vi "Process.vi"(8 "error in":errorcluster, 11 "GUI":refnum<class "GUI.lvclass">) -> (0 "error out":errorcluster, 3 "GUI out":refnum<class "GUI.lvclass">)   [LabVIEW 2022 SP3, in "GUI.lvclass"]
doc: "---------------------------------------------------------------\nJKI State Machine Objects™\nhttp://jki.net/state-machine-objects/\nCopyright (C) 2005-2015, JKI <info@jki.net>\nALL RIGHTS RESERVEDJKI State Machine Objects (SMO) 1.0.0.5\nJKI - JKI\nCopyright (c) 2016, JKI"
uses:
  GUI.lvclass
  <vilib>/JKI/JKI SMO/SMO/SMO.lvclass
  <vilib>/JKI/JKI SMO/SMO/Typedefs/Parent Call--Enum.ctl
  Typedefs/Value.ctl
  <vilib>/JKI/JKI SMO/SMO.UI/SMO.UI.lvclass
  DB2/DB2.lvclass
  Analyzer/Analyzer.lvclass
  Home/Home.lvclass
  C:/Program Files (x86)/National Instruments/LabVIEW 2022/vi.lib/JKI/JKI SMO/SMO.UI/SMO.UI.lvclass
  C:/Program Files (x86)/National Instruments/LabVIEW 2022/vi.lib/JKI/JKI SMO/SMO/SMO.lvclass
  C:/Users/uib01493/Documents/CIS_580_Data_Analytics_in_SW_Eng/002_Source_Code/002_GUI/002_SRC/GUI/GUI.lvclass
panel:
  in  "Menu Btns":T1(radio) caption="Radio Btns"
  out "Status":string
  # "Software Requirements Tracing Tool (development)"
  # "For instructions on how to use the JKI State Machine Objects, examples and video tutorials, visit:\nhttp://jki.net/state-machine-objects/\n\nJKI State Machine Objects™\nhttp://jki.net/state-machine-objects/\nCopyright (C) 2005-2015, JKI <info@jki.net>\nALL RIGHTS RESERVED"
types:
  T1 = enum32{"Home", "Analyzer", "Button 3", "Settings"}
  T2 = typedef "SMO.lvclass/Parent Call--Enum.ctl" = enum16{"Allows parent to run", "Does not request parent to run"}
  T3 = enum32{"invalid app kind", "Development System", "Run Time System", "Student Edition", "Embedded LabVIEW", "Evaluation", "Custom"}
  T4 = enum32{"Invalid", "Standard", "Closed", "Hidden", "Minimized", "Maximized"}
  T5 = typedef "GUI.lvclass/Value.ctl" = string
  T6 = cluster{"Core":cluster{"Current VI Reference":refnum<vi>, "Close Panel on Exit?":bool, "error":errorcluster}, "Self Reference":refnum<class "GUI.lvclass">, "Value":T5, "Sub Panel":refnum<vi>, "Status":string, "NewSettingsConfig":cluster{"Requirements Definition (.csv)":path, "Report Generation Save Path":path, "Source Code to Analyze":path, "Search By:":string, "Word/Phrase:":string}}
  T7 = cluster{"Requirements Definition (.csv)":path, "Report Generation Save Path":path, "Source Code to Analyze":path, "Search By:":string, "Word/Phrase:":string}
  T8 = cluster{"Current VI Reference":refnum<vi>, "Close Panel on Exit?":bool, "error":errorcluster}
  T9 = typedef "GUI.lvclass/PrivateEvents--Cluster.ctl" = cluster{"New Value":refnum<user-event>}
  T10 = typedef "SMO.lvclass/Protected Events.ctl" = cluster{"StopProcesses":refnum<user-event>, "AbortProcesses":refnum<user-event>, "Config Changed":refnum<user-event>, "Dependency":refnum<user-event>}
  T11 = typedef "Home.lvclass/PublicEvents--Cluster.ctl" = cluster{"UI State":refnum<user-event>}
  T12 = typedef "Analyzer.lvclass/PublicEvents--Cluster.ctl" = cluster{"UI State":refnum<user-event>, "NewEventMessage":refnum<user-event>}
  T13 = typedef "DB2.lvclass/PublicEvents--Cluster.ctl" = cluster{"UI State":refnum<user-event>, "NewSettingsConfig":refnum<user-event>}
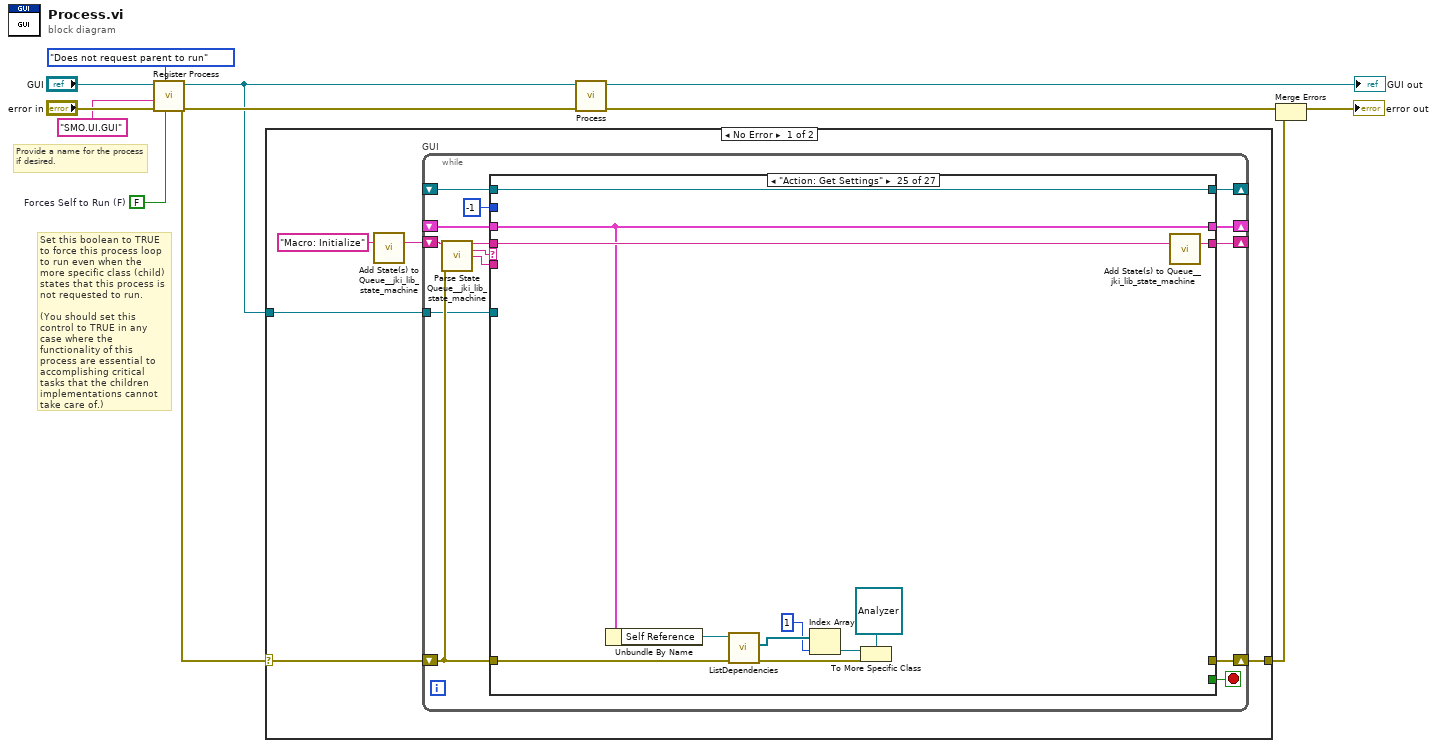
[diagram p0: block diagram]
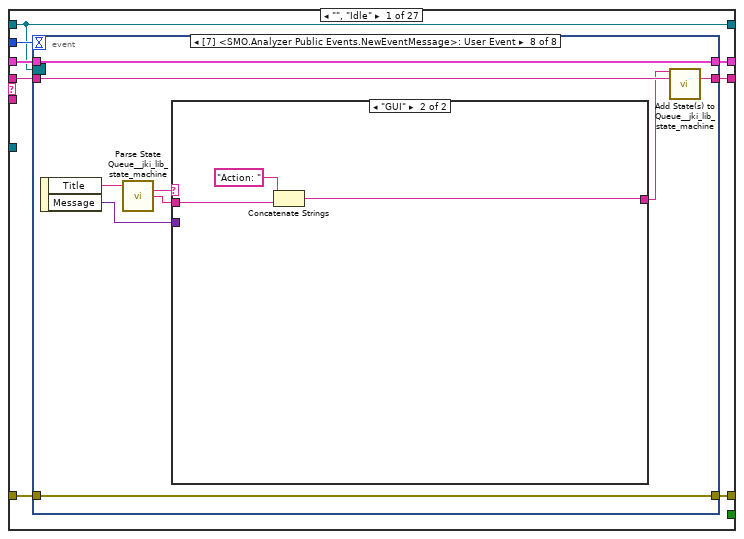
[diagram p2: hidden frame]
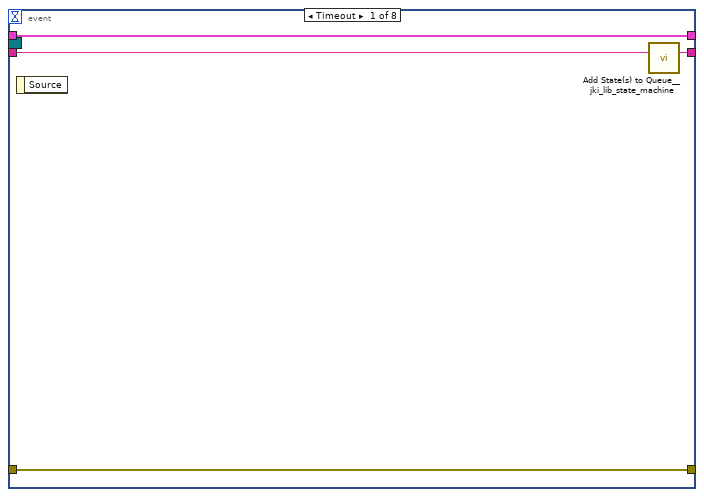
[diagram p3: hidden frame]
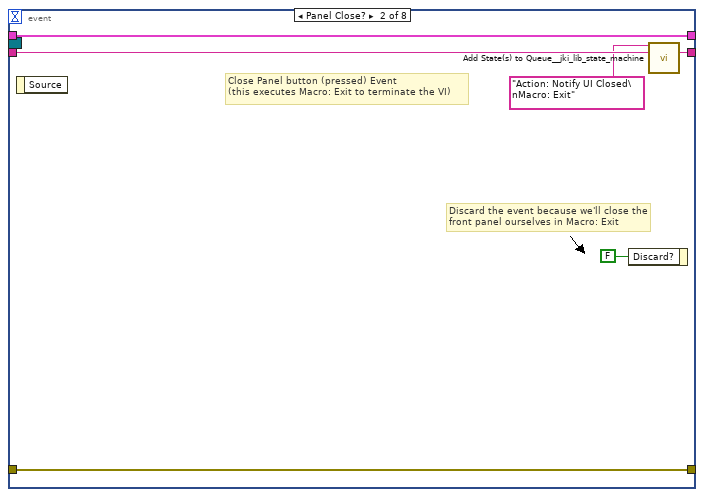
[diagram p4: hidden frame]
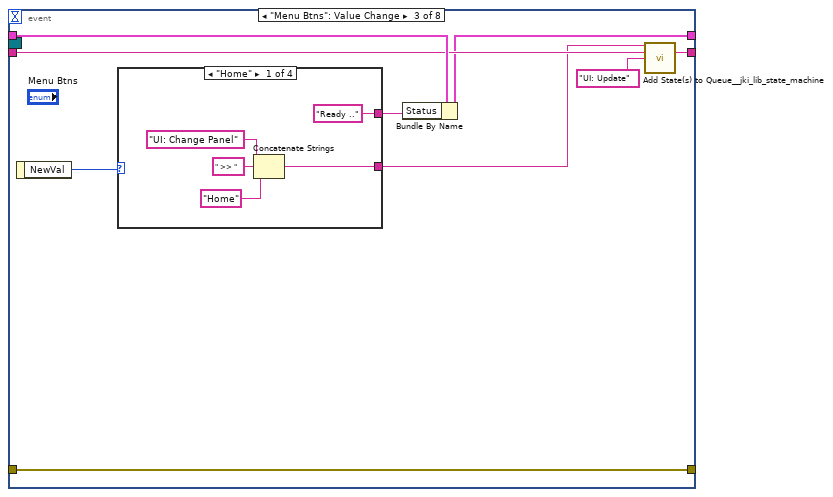
[diagram p5: hidden frame]
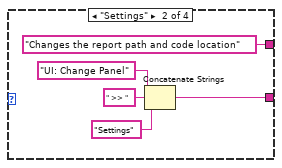
[diagram p6: hidden frame]
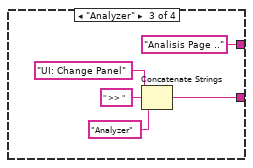
[diagram p7: hidden frame]
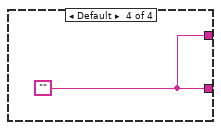
[diagram p8: hidden frame]
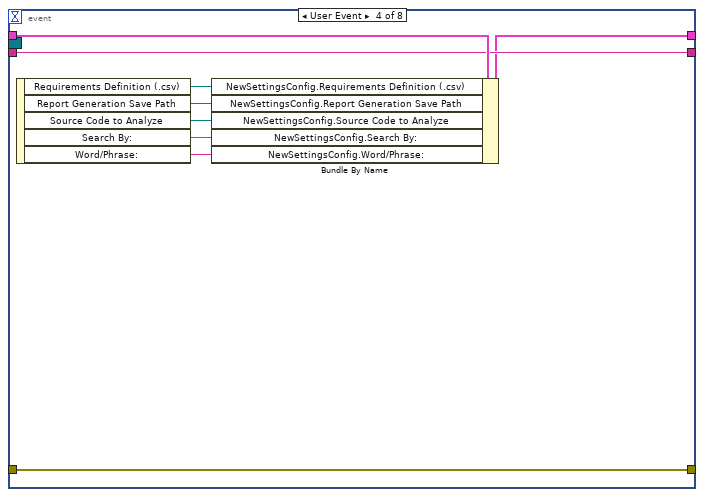
[diagram p9: hidden frame]
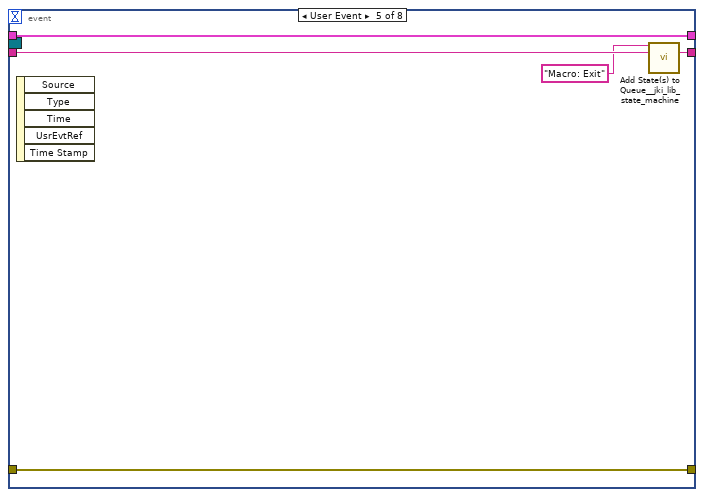
[diagram p10: hidden frame]
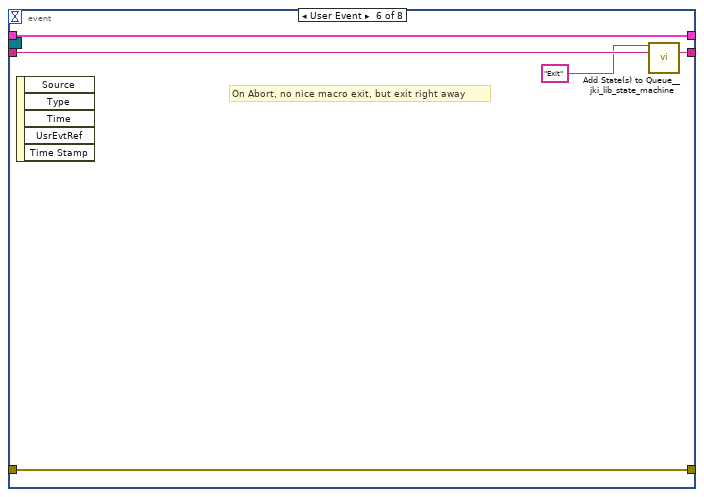
[diagram p11: hidden frame]
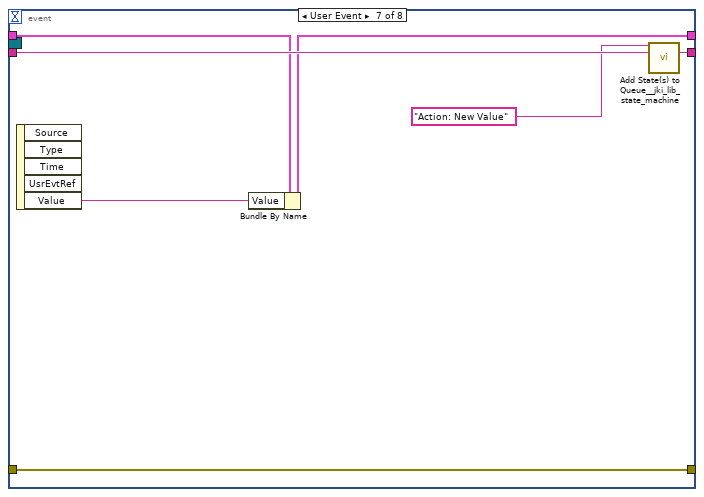
[diagram p12: hidden frame]
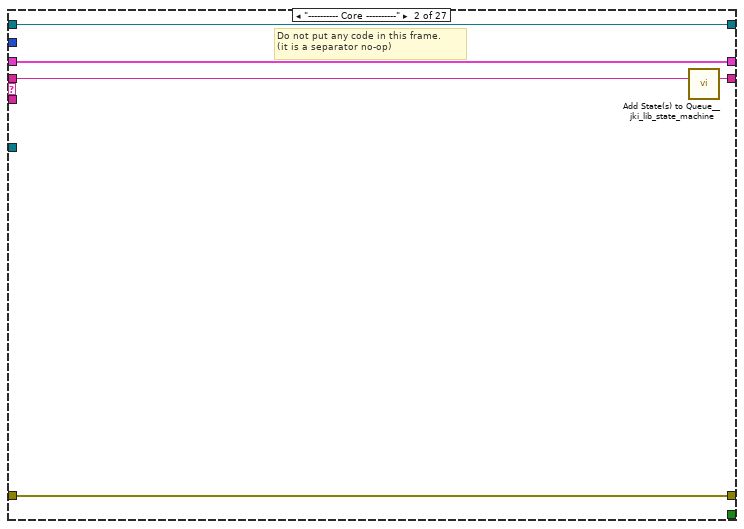
[diagram p14: hidden frame]
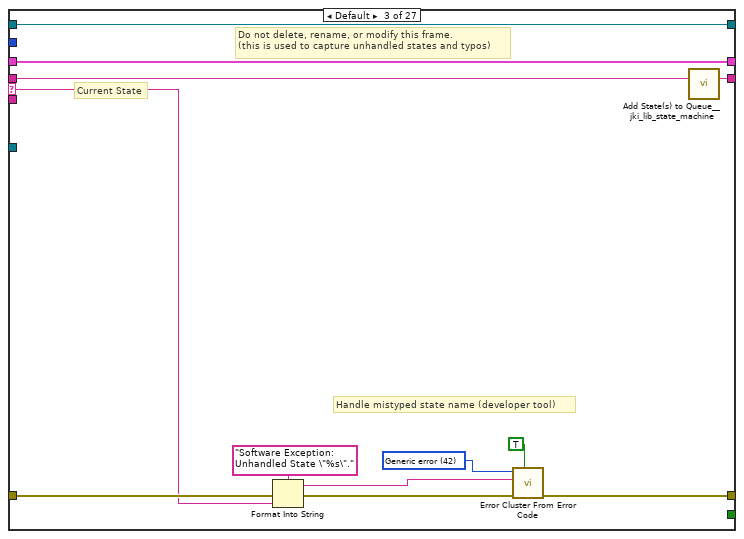
[diagram p15: hidden frame]
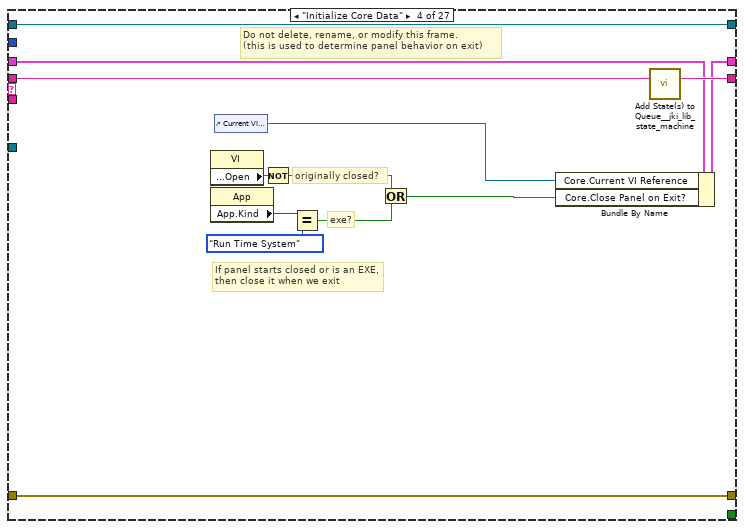
[diagram p16: hidden frame]
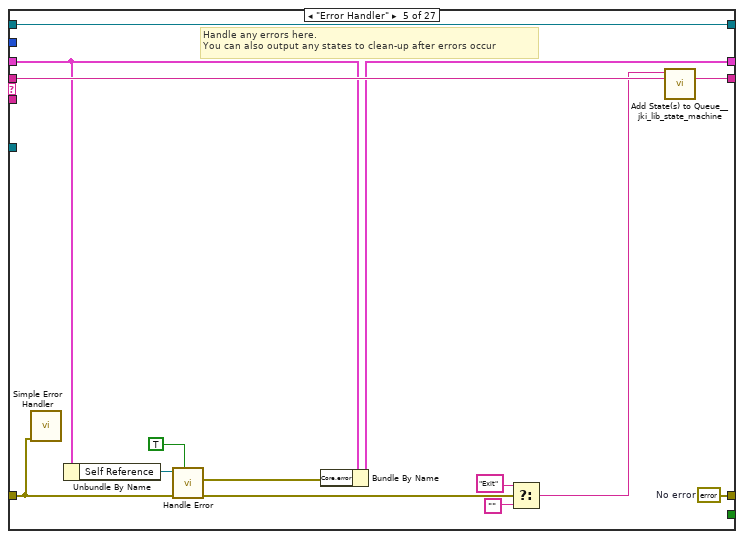
[diagram p17: hidden frame]
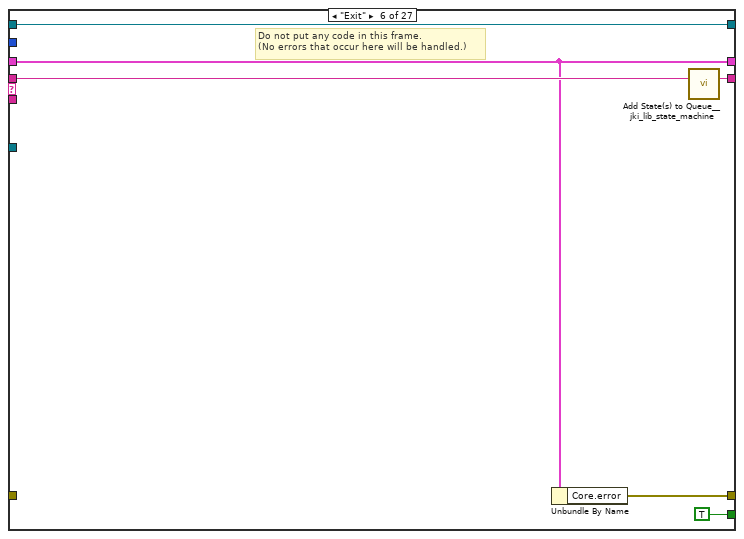
[diagram p18: hidden frame]
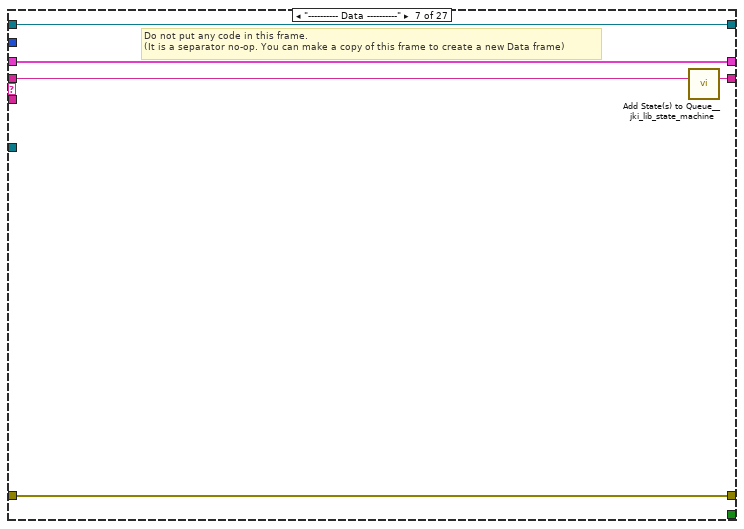
[diagram p19: hidden frame]
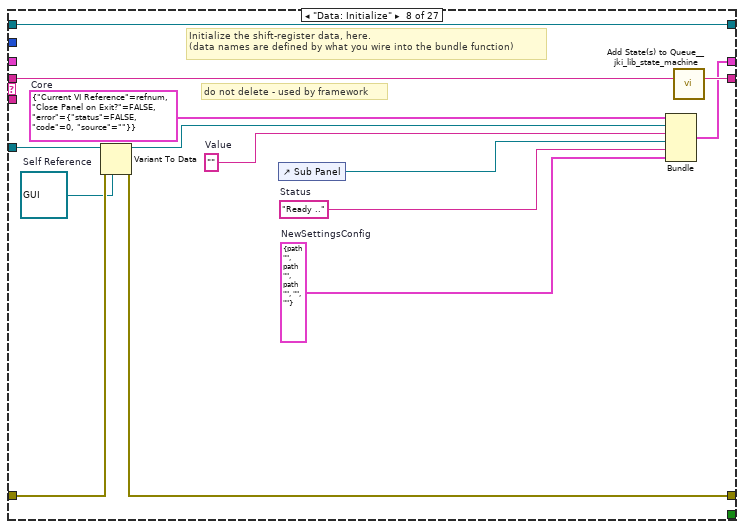
[diagram p20: hidden frame]
diagram:
  w2 = FALSE  # Forces Self to Run (F)
  # "Provide a name for the process\nif desired."
  # "Set this boolean to TRUE to force this process loop to run even when the more specific class (child) states that this process is not requested to run.\n\n(You should set this control to TRUE in any case where the functionality of this process are essential to accomplishing critical tasks that the children implementations cannot take care of.)"
  n1 = call <vilib>:"Register Process.vi"("Forces Self to Run (F)"=w2, "Parent Call"=Parent_Call--Enum."Does not request parent to run", "error in (no error)"="error in", "Process Name (optional)"="SMO.UI.GUI", "SMO"="GUI") -> ("error out"=w8:errorcluster, "SMO out"=w7:refnum<class "GUI.lvclass">)  [unwired: 5 in]
  n2 = case shown="No Error" w8 {
    selector: w8 -> [w13 w412]
    tunnel: w7 -> [w14 _]
    tunnel: [w12 w412] -> w4
    frame No Error {
      n3 = call <vilib>:"Add State(s) to Queue__jki_lib_state_machine.vi"("State(s) in (\"\")"="Macro: Initialize") -> ("States Out"=w16:string)  [unwired: 14 in]
      n4 = while "GUI" {
        shift-right: [w23] -> _
        shift-left: _ -> [w22]
        shift-right: [w26] -> w12
        shift-left: w13 -> [w20]
        shift-right: [w25] -> _
        shift-left: w16 -> [w27]
        tunnel: w14 -> [w19]
        shift-right: [w18] -> _
        shift-left: _ -> [w17]
        stop <- w24 stop-if-true
        n5 = call <vilib>:"Parse State Queue__jki_lib_state_machine.vi"("State Queue"=w27, "Error In (no error)"=w20) -> ("Remaining States"=w29:string, "Current State"=w30:string, "Arguments"=w28:string)  [unwired: 11 in]
        n6 = case shown="\"Action: Get Settings\"" w30 {
          selector: w30 -> [_ _ w118 _ _ _ _ _ _ _ _ _ _ _ _ _ _ _ _ _ _ _ _ _ _ _ _]
          tunnel: w29 -> [w38 w116 w122 w141 w155 w161 w166 w180 w187 w192 w198 w204 w211 w227 w260 w301 w310 w324 w329 w340 w345 w374 w380 w385 w396 w404 w411]
          tunnel: w28 -> [_ _ _ _ _ _ _ _ _ _ _ _ w205 w221 w256 _ _ _ _ _ _ _ _ _ _ _ _]
          tunnel: w22 -> [w36 w113 w120 w132 w145 w157 w163 _ w183 w189 w194 w200 w209 w223 w255 w298 w306 w315 w326 w337 w342 w372 w378 w383 w393 w401 w408]
          tunnel: [w35 w114 w124 w138 w147 w156 w164 w170 w184 w190 w195 w202 w206 w224 w257 w299 w308 w322 w327 w331 w343 w364 w376 w381 _ w397 w405] -> w26
          tunnel: w20 -> [w34 w114 w123 w138 w142 _ w164 w177 w181 w190 w195 w202 w207 w225 w258 w299 w308 w322 w327 w332 w343 w367 w376 w381 w386 w398 w406]
          tunnel: [w37 w115 w121 w140 w154 w160 w165 w179 w186 w191 w197 w203 w210 w226 w260 w300 w309 w323 w328 w339 w344 w373 w379 w384 w395 w403 w410] -> w25
          tunnel: [_ _ _ _ _ TRUE _ _ _ _ _ _ _ _ _ _ _ _ _ _ _ _ _ _ _ _ _] -> w24
          tunnel: [w33 w113 w120 w139 w144 w157 w163 w178 w183 w189 w194 w200 w209 w223 w255 w298 w306 w315 w326 w337 w342 w372 w378 w383 w393 w401 w408] -> w23
          tunnel: -1 ("Timeout") -> [w32 _ _ _ _ _ _ _ _ _ _ _ _ _ _ _ _ _ _ _ _ _ _ _ _ _ _]
          tunnel: w19 -> [_ _ _ _ _ _ _ w175 _ _ _ _ _ _ _ _ _ _ _ _ _ _ _ _ _ _ _]
          tunnel: [w31 w112 w117 w129 w153 w158 w162 w173 w182 w188 w196 w201 w208 w220 w259 w297 w307 w316 w325 w338 w341 w371 w377 w382 w394 w402 w409] -> w18
          tunnel: w17 -> [w31 w112 w117 w129 w153 w158 w162 w173 w182 w188 w196 w201 w208 w220 w259 w297 w307 w316 w325 w338 w341 _ w377 w382 w394 w402 w409]
          frame "", "Idle" {
            n7 = event shown="[7] <SMO.Analyzer Public Events.NewEventMessage>: User Event" {
              selector: w31 -> [_ _ _ _ _ _ _ _]
              dyn-events: _ -> [_ _ _ _ _ _ _ _]
              timeout: w32 -> [_ _ _ _ _ _ _ _]
              tunnel: w38 -> [w42 w48 w54 w81 w87 w92 w99 w101]
              tunnel: [w41 w47 w55 w81 w86 w91 w98 w102] -> w37
              tunnel: w36 -> [w39 w45 w57 w82 w84 w89 w95 w108]
              tunnel: [w40 w46 w56 w80 w85 w90 w97 w107] -> w35
              tunnel: w34 -> [w40 w46 w56 w80 w85 w90 w97 w107]
              tunnel: [w39 w45 w51 w79 w84 w89 w94 w108] -> w33
              event Timeout {
                n8 = event-data() -> ()  [unwired: 1 in, 1 out]
                n9 = call <vilib>:"Add State(s) to Queue__jki_lib_state_machine.vi"("State(s) in (\"\")"=w42) -> ("States Out"=w41:string)  [unwired: 14 in]
              }
              event Panel Close? {
                # "Discard the event because we'll close the front panel ourselves in Macro: Exit"
                # "Close Panel button (pressed) Event\n(this executes Macro: Exit to terminate the VI)"
                n10 = event-data() -> ()  [unwired: 1 in, 1 out]
                n11 = event-data("Discard?"=FALSE) -> ()  [unwired: 1 in, 1 out]
                n12 = call <vilib>:"Add State(s) to Queue__jki_lib_state_machine.vi"("State(s) in Front (\"\")"="Action: Notify UI Closed\nMacro: Exit", "State(s) in (\"\")"=w48) -> ("States Out"=w47:string)  [unwired: 13 in]
              }
              event "Menu Btns": Value Change {
                n13 = event-data() -> ("NewVal"=w53:T1)  [unwired: 1 in]
                n14 = case shown="\"Home\"" w53 {
                  tunnel: [w61 w66 w68 w73] -> w52
                  tunnel: ["Ready .." "Changes the report path and code location" "Analisis Page .." w73] -> w50
                  frame "Home" {
                    n15 = Concatenate Strings("UI: Change Panel", " >> " ("string"), "Home") -> (w61:string)
                  }
                  frame "Settings" {
                    n16 = Concatenate Strings("UI: Change Panel", " >> " ("string"), "Settings") -> (w66:string)
                  }
                  frame "Analyzer" {
                    n17 = Concatenate Strings("UI: Change Panel", " >> " ("string"), "Analyzer") -> (w68:string)
                  }
                  frame Default {
                    w73 = ""
                  }
                }
                n18 = Bundle By Name(cluster=w57, "Status"=w50) -> (w51:T6)
                n19 = call <vilib>:"Add State(s) to Queue__jki_lib_state_machine.vi"("State(s) in Front (\"\")"=w52, "State(s) in (\"\")"=w54, "State(s) at Back (\"\")"="UI: Update" ("State(s) at Back (\"\")")) -> ("States Out"=w55:string)  [unwired: 12 in]
              }
              event User Event {
                n20 = event-data() -> ("Requirements Definition (.csv)"=w78:path, "Report Generation Save Path"=w77:path, "Source Code to Analyze"=w76:path, "Search By:"=w75:string, "Word/Phrase:"=w74:string)  [unwired: 1 in]
                n21 = Bundle By Name(cluster=w82, "NewSettingsConfig.Requirements Definition (.csv)"=w78, "NewSettingsConfig.Report Generation Save Path"=w77, "NewSettingsConfig.Source Code to Analyze"=w76, "NewSettingsConfig.Search By:"=w75, "NewSettingsConfig.Word/Phrase:"=w74) -> (w79:T6)
              }
              event User Event {
                n22 = event-data() -> ()  [unwired: 1 in, 5 out]
                n23 = call <vilib>:"Add State(s) to Queue__jki_lib_state_machine.vi"("State(s) in Front (\"\")"="Macro: Exit", "State(s) in (\"\")"=w87) -> ("States Out"=w86:string)  [unwired: 13 in]
              }
              event User Event {
                # "On Abort, no nice macro exit, but exit right away"
                n24 = event-data() -> ()  [unwired: 1 in, 5 out]
                n25 = call <vilib>:"Add State(s) to Queue__jki_lib_state_machine.vi"("State(s) in Front (\"\")"="Exit", "State(s) in (\"\")"=w92) -> ("States Out"=w91:string)  [unwired: 13 in]
              }
              event User Event {
                n26 = event-data() -> ("Value"=w96:string)  [unwired: 1 in, 4 out]
                n27 = Bundle By Name(cluster=w95, "Value"=w96) -> (w94:T6)
                n28 = call <vilib>:"Add State(s) to Queue__jki_lib_state_machine.vi"("State(s) in Front (\"\")"="Action: New Value", "State(s) in (\"\")"=w99) -> ("States Out"=w98:string)  [unwired: 13 in]
              }
              event User Event {
                n29 = event-data() -> ("Title"=w106:string, "Message"=w103:variant)  [unwired: 1 in]
                n30 = call <vilib>:"Parse State Queue__jki_lib_state_machine.vi"("State Queue"=w106) -> ("Current State"=w105:string, "Arguments"=w104:string)  [unwired: 12 in, 1 out]
                n31 = case shown="\"GUI\"" w105 {
                  tunnel: w104 -> [_ w110]
                  tunnel: w103 -> [_ _]
                  tunnel: [_ w109] -> w100
                  frame Default {
                  }
                  frame "GUI" {
                    n32 = Concatenate Strings("Action: ", w110) -> (w109:string)
                  }
                }
                n33 = call <vilib>:"Add State(s) to Queue__jki_lib_state_machine.vi"("State(s) in Front (\"\")"=w100, "State(s) in (\"\")"=w101) -> ("States Out"=w102:string)  [unwired: 13 in]
              }
            }
          }
          frame "---------- Core ----------" {
            # "Do not put any code in this frame.\n(it is a separator no-op)"
            n34 = call <vilib>:"Add State(s) to Queue__jki_lib_state_machine.vi"("State(s) in (\"\")"=w116) -> ("States Out"=w115:string)  [unwired: 14 in]
          }
          frame Default {
            w127 = 42 items=["No error", "Argument error", "Memory is full", "Out of zone", "End of file", "File already open", "Generic file I/O error", "File not found", "File permission error", "Disk is full", "Duplicate path", "Too many files open", "System feature not enabled", "Resource file not found", "Cannot add resource", "Resource not found", "Image not found", "Image memory error", "Pen does not exist", "Config type invalid", "Config token not found", "Config parse error", "Config memory error", "Bad external code format", "Bad external code offset", "External code not present", "Null window", "Destroy window error", "Null menu", "Print aborted", "Bad print record", "Print driver error", "Windows error during printing", "Memory error during printing", "Print dialog error", "Generic print error", "Invalid device refnum", "Device not found", "Device parameter error", "Device unit error", "Cannot open device", "Device call aborted", "Generic error", "Cancelled by user", "Object ID too low", "Object ID too high", "Object not in heap", "Unknown heap", "Unknown object (invalid DefProc)", "Unknown object (DefProc not in table)", "Message out of range", "Invalid (null) method", "Unknown message", "Manager call not supported", "Bad address", "Network operation in progress", "Network operation timed out", "Connection is busy", "Network attribute not supported", "Network error", "Address in use", "System out of memory", "Connection aborted", "Connection refused", "Not connected", "Already connected", "Connection closed", "Initialization error (interapplication manager)", "Bad occurrence", "Wait on unbound occurrence handler", "Occurrence queue overflow", "Datalog type conflict", "Unused", "Unrecognized type (interapplication manager)", "Memory corrupt", "Failed to make temporary DLL", "Old CIN version", "Drag socket not found", "Failed to load drop-object", "Failed to register OLE object", "Failed to release OLE object", "Format specifier type mismatch", "Unknown format specifier", "Too few format specifiers", "Too many format specifiers", "Scan failed", "Newer CIN version", "Error converting to variant", "Runtime menu error", "Password tampered", "Variant attribute not found", "Incompatible variant data type", "Event data is not available", "Event Store is not present", "Occurrence is not found", "Event Queue is not created", "Event info is not available", "Refnum passed is NULL", "Error retrieving Class GUID", "Error retrieving CoClass GUID", "Error retrieving TypeLib GUID.", "Bad built application magic bytes.", "Specific driver is different from the specific driver associated with the Logical Name.", "There is no session opened to the class driver.", "Max Error", "MAX - Error with config objects", "MAX - Error loading configuration", "MAX - Group not supported"]
            # "Current State"
            # "Do not delete, rename, or modify this frame.\n(this is used to capture unhandled states and typos)"
            # "Handle mistyped state name (developer tool)"
            n35 = Format Into String(format string="Software Exception: Unhandled State \"%s\"." ("message"), error in=w123, w118) -> (resulting string=w126:string, error out=w125:errorcluster)  [unwired: 1 in]
            n36 = call <vilib>:"Error Cluster From Error Code.vi"("show call chain? (False)"=TRUE, "error in (no error)"=w125, "error message (\"\")"=w126, "error code (0)"=w127) -> ("error out"=w124:errorcluster)  [unwired: 5 in]
            n37 = call <vilib>:"Add State(s) to Queue__jki_lib_state_machine.vi"("State(s) in (\"\")"=w122) -> ("States Out"=w121:string)  [unwired: 14 in]
          }
          frame "Initialize Core Data" {
            # "Do not delete, rename, or modify this frame.\n(this is used to determine panel behavior on exit)"
            # "originally closed?"
            # "exe?"
            # "If panel starts closed or is an EXE, then close it when we exit"
            n38 = property class="VI"() -> ("Front Panel.Open"=w137:bool)  [unwired: 2 in, 2 out]
            n39 = property class="App"() -> ("App.Kind"=w136:T3)  [unwired: 2 in, 2 out]
            n40 = control-ref of="Current VI Reference"() -> (w130:refnum<vi>)
            n41 = Not(x=w137) -> (.not. x?=w134:bool)
            n42 = Equal?(x=w136, y=T3."Run Time System" ("Application:Kind")) -> (x = y?=w133:bool)
            n43 = Or(x=w134, y=w133) -> (x .or. y?=w131:bool)
            n44 = Bundle By Name(cluster=w132, "Core.Current VI Reference"=w130, "Core.Close Panel on Exit?"=w131) -> (w139:T6)
            n45 = call <vilib>:"Add State(s) to Queue__jki_lib_state_machine.vi"("State(s) in (\"\")"=w141) -> ("States Out"=w140:string)  [unwired: 14 in]
          }
          frame "Error Handler" {
            w147 = errorcluster {"status"=FALSE, "code"=0, "source"=""}  # No error
            # "Handle any errors here.\nYou can also output any states to clean-up after errors occur"
            n46 = call <vilib>:"Simple Error Handler.vi"("error in (no error)"=w142) -> ()  [unwired: 4 in, 5 out]
            n47 = Unbundle By Name(w145) -> ("Self Reference"=w152:refnum<class "GUI.lvclass">)
            n48 = call-dynamic "Handle Error.vi"("Stop on Unhandled Error (T)"=TRUE, "error in"=w142, "GUI"=w152) -> ("handling error"=w148:errorcluster, "Unhandled error"=w146:errorcluster)  [unwired: 6 in, 1 out]
            n49 = Bundle By Name(cluster=w145, "Core.error"=w146) -> (w144:T6)
            n50 = Select(t="Exit", s=w148, f="") -> (s? t:f=w149:string)
            n51 = call <vilib>:"Add State(s) to Queue__jki_lib_state_machine.vi"("State(s) in Front (\"\")"=w149, "State(s) in (\"\")"=w155) -> ("States Out"=w154:string)  [unwired: 13 in]
          }
          frame "Exit" {
            # "Do not put any code in this frame.\n(No errors that occur here will be handled.)"
            n52 = Unbundle By Name(w157) -> ("Core.error"=w156:errorcluster)
            n53 = call <vilib>:"Add State(s) to Queue__jki_lib_state_machine.vi"("State(s) in (\"\")"=w161) -> ("States Out"=w160:string)  [unwired: 14 in]
          }
          frame "---------- Data ----------" {
            # "Do not put any code in this frame.\n(It is a separator no-op. You can make a copy of this frame to create a new Data frame)"
            n54 = call <vilib>:"Add State(s) to Queue__jki_lib_state_machine.vi"("State(s) in (\"\")"=w166) -> ("States Out"=w165:string)  [unwired: 14 in]
          }
          frame "Data: Initialize" {
            w167 = T7 {"Requirements Definition (.csv)"=path "", "Report Generation Save Path"=path "", "Source Code to Analyze"=path "", "Search By:"="", "Word/Phrase:"=""}  # NewSettingsConfig
            w168 = "Ready .."  # Status
            w171 = T5 ""  # Value
            w172 = T8 {"Current VI Reference"=refnum, "Close Panel on Exit?"=FALSE, "error"={"status"=FALSE, "code"=0, "source"=""}}  # Core
            w176 = refnum<class "GUI.lvclass"> refnum  # Self Reference
            # "do not delete - used by framework"
            # "Initialize the shift-register data, here.\n(data names are defined by what you wire into the bundle function)"
            n55 = Variant To Data(error in=w177, type=w176, Variant=w175) -> (data=w174:refnum<class "GUI.lvclass">, error out=w170:errorcluster)
            n56 = control-ref of="Sub Panel"() -> (w169:refnum<vi>)
            n57 = Bundle("Core"=w172, "Self Reference"=w174, "Value"=w171, "Sub Panel"=w169, "Status"=w168, "NewSettingsConfig"=w167) -> (w178:T6)  [unwired: 1 in]
            n58 = call <vilib>:"Add State(s) to Queue__jki_lib_state_machine.vi"("State(s) in (\"\")"=w180) -> ("States Out"=w179:string)  [unwired: 14 in]
          }
          frame "Data: Cleanup" {
            # "Cleanup any data and references, here.\n(this is called automatically, by the Macro: Exit)"
            n59 = Unbundle By Name(w183) -> ("Core.Current VI Reference"=w185:refnum<vi>)
            n60 = Close Reference(reference=w185, error in (no error)=w181) -> (error out=w184:errorcluster)
            n61 = call <vilib>:"Add State(s) to Queue__jki_lib_state_machine.vi"("State(s) in (\"\")"=w187) -> ("States Out"=w186:string)  [unwired: 14 in]
          }
          frame "---------- UI ----------" {
            # "Do not put any code in this frame.\n(It is a separator no-op. You can make a copy of this frame to create a new UI frame)"
            n62 = call <vilib>:"Add State(s) to Queue__jki_lib_state_machine.vi"("State(s) in (\"\")"=w192) -> ("States Out"=w191:string)  [unwired: 14 in]
          }
          frame "UI: Initialize" {
            # "Initialize the User Interface, here.\n(this is called automatically, by the Macro: Init)"
            n63 = control-ref of="This VI"() -> (w193:refnum<vi>)
            n64 = invoke class="VI" method="Default Vals.Reinit All"(reference=w193) -> ()  [unwired: 2 in, 3 out]
            n65 = call <vilib>:"Add State(s) to Queue__jki_lib_state_machine.vi"("State(s) in (\"\")"=w198) -> ("States Out"=w197:string)  [unwired: 14 in]
          }
          frame "UI: Update" {
            # "Do not put any code in this frame.\n(It is a separator no-op. You can make a copy of this frame to create a new UI frame)"
            n66 = Unbundle By Name(w200) -> ("Status"=→"Status":string)
            n67 = call <vilib>:"Add State(s) to Queue__jki_lib_state_machine.vi"("State(s) in (\"\")"=w204) -> ("States Out"=w203:string)  [unwired: 14 in]
          }
          frame "UI: Cursor Set" {
            # "Argument"
            # "Initialize the User Interface, here.\n(this is called automatically, by the Macro: Init)"
            n68 = disable-structure shown="Default" {
              disable-tunnel: w207 -> [w212 w215]
              disable-tunnel: [w212 w214] -> w206
              disable-tunnel: w205 -> [_ w213]
              frame condition #0 {
              }
              frame condition #1 (active) {
                n69 = case shown="\"Idle\", Default" w213 {
                  tunnel: w215 -> [w217 w219]
                  tunnel: [w216 w218] -> w214
                  frame "Idle", Default {
                    n70 = call <vilib>:"Unset Busy.vi"("error in (no error)"=w217) -> ("error out"=w216:errorcluster)  [unwired: 10 in]
                  }
                  frame "Busy" {
                    n71 = call <vilib>:"Set Busy.vi"("error in (no error)"=w219) -> ("error out"=w218:errorcluster)  [unwired: 9 in, 1 out]
                  }
                }
              }
            }
            n72 = call <vilib>:"Add State(s) to Queue__jki_lib_state_machine.vi"("State(s) in (\"\")"=w211) -> ("States Out"=w210:string)  [unwired: 14 in]
          }
          frame "UI: Front Panel State" {
            # "Argument"
            # "Set Front Panel Open or Closed\n(Usage: \"UI: Front Panel State >> Open|Close\")"
            n73 = Unbundle By Name(w223) -> ("Core.Current VI Reference"=w222:refnum<vi>)
            n74 = disable-structure shown="Default" {
              disable-tunnel: w225 -> [w231 w254]
              disable-tunnel: [w230 w254] -> w224
              disable-tunnel: w222 -> [w229 _]
              disable-tunnel: w221 -> [w228 _]
              frame condition #0 (active) {
                n75 = case shown="\"Open\", Default" w228 {
                  tunnel: w231 -> [w235 w248]
                  tunnel: [w237 w249] -> w230
                  tunnel: w229 -> [w236 w246]
                  frame "Open", Default {
                    n76 = property class="VI"(reference=w236, error in=w235) -> (reference out=w233:refnum<vi>, error out=w234:errorcluster, "FP.State"=w232:T4)
                    n77 = case shown="\"Closed\"" w232 {
                      tunnel: [w240 w243] -> w237
                      tunnel: w234 -> [w239 w243]
                      tunnel: w233 -> [w238 _]
                      frame "Closed" {
                        n78 = invoke class="VI" method="FP.Open"(reference=w238, error in=w239, "Activate"=TRUE, "State"=T4."Standard") -> (error out=w240:errorcluster)  [unwired: 1 in, 4 out]
                      }
                      frame Default {
                      }
                    }
                  }
                  frame "Close" {
                    n79 = property class="VI"(reference=w246, error in=w248) -> (reference out=w245:refnum<vi>, error out=w247:errorcluster, "FP.State"=w244:T4)
                    n80 = case shown="Default" w244 {
                      tunnel: [w250 w253] -> w249
                      tunnel: w247 -> [w250 w252]
                      tunnel: w245 -> [_ w251]
                      frame "Invalid", "Closed" {
                      }
                      frame Default {
                        n81 = invoke class="VI" method="FP.Close"(reference=w251, error in=w252) -> (error out=w253:errorcluster)  [unwired: 1 in, 2 out]
                      }
                    }
                  }
                }
              }
              frame condition #1 {
              }
            }
            n82 = call <vilib>:"Add State(s) to Queue__jki_lib_state_machine.vi"("State(s) in (\"\")"=w227) -> ("States Out"=w226:string)  [unwired: 14 in]
          }
          frame "UI: Change Panel" {
            n83 = case shown="\"Settings\"" w256 {
              tunnel: w258 -> [w261 w264 w280 w292]
              tunnel: [w261 w263 w276 w288] -> w257
              tunnel: w255 -> [_ w272 w279 w291]
              frame Default {
              }
              frame "Settings" {
                n84 = Unbundle By Name(w272) -> ("Sub Panel"=w268:refnum<vi>, "Self Reference"=w267:refnum<class "GUI.lvclass">)
                n85 = call <vilib>:"ListDependencies.vi"("error in (no error)"=w264, "SMO in"=w267) -> ("error out"=w265:errorcluster, "[Dependencies]"=w271:refnum<class "SMO.lvclass">[])  [unwired: 6 in, 2 out]
                n86 = Index Array(array=w271) -> (element=w270:refnum<class "SMO.lvclass">)  [unwired: 1 in]
                n87 = To More Specific Class(target class=refnum<class "DB2.lvclass"> refnum ("DB2.lvclass"), reference=w270, error in=w265) -> (specific class reference=w262:refnum<class "DB2.lvclass">, error out=w266:errorcluster)
                n88 = call "Show.vi"("Subpanel Ref (empty: open detached)"=w268, "error in (no error)"=w266, "DB2"=w262) -> ("error out"=w263:errorcluster)  [unwired: 7 in, 1 out]
              }
              frame "Analyzer" {
                n89 = Unbundle By Name(w279) -> ("Sub Panel"=w274:refnum<vi>, "Self Reference"=w282:refnum<class "GUI.lvclass">)
                n90 = call <vilib>:"ListDependencies.vi"("error in (no error)"=w280, "SMO in"=w282) -> ("error out"=w281:errorcluster, "[Dependencies]"=w284:refnum<class "SMO.lvclass">[])  [unwired: 6 in, 2 out]
                n91 = Index Array(array=w284, index=1) -> (element=w283:refnum<class "SMO.lvclass">)
                n92 = To More Specific Class(target class=refnum<class "Analyzer.lvclass"> refnum ("Analyzer.lvclass"), reference=w283, error in=w281) -> (specific class reference=w273:refnum<class "Analyzer.lvclass">, error out=w275:errorcluster)
                n93 = call "Show.vi"("Subpanel Ref (empty: open detached)"=w274, "error in (no error)"=w275, "Analyzer"=w273) -> ("error out"=w276:errorcluster)  [unwired: 7 in, 1 out]
              }
              frame "Home" {
                n94 = Unbundle By Name(w291) -> ("Sub Panel"=w286:refnum<vi>, "Self Reference"=w294:refnum<class "GUI.lvclass">)
                n95 = call <vilib>:"ListDependencies.vi"("error in (no error)"=w292, "SMO in"=w294) -> ("error out"=w293:errorcluster, "[Dependencies]"=w296:refnum<class "SMO.lvclass">[])  [unwired: 6 in, 2 out]
                n96 = Index Array(array=w296, index=2) -> (element=w295:refnum<class "SMO.lvclass">)
                n97 = To More Specific Class(target class=refnum<class "Home.lvclass"> refnum ("Home.lvclass"), reference=w295, error in=w293) -> (specific class reference=w285:refnum<class "Home.lvclass">, error out=w287:errorcluster)
                n98 = call "Show.vi"("Subpanel Ref (empty: open detached)"=w286, "error in (no error)"=w287, "Home"=w285) -> ("error out"=w288:errorcluster)  [unwired: 7 in, 1 out]
              }
            }
          }
          frame "---------- Macro ----------" {
            # "Do not put any code in this frame.\n(It is a separator no-op. You can make a copy of this frame to create a new Macro frame)"
            n99 = call <vilib>:"Add State(s) to Queue__jki_lib_state_machine.vi"("State(s) in (\"\")"=w301) -> ("States Out"=w300:string)  [unwired: 14 in]
          }
          frame "Macro: Initialize" {
            w304 = "UI: Initialize\nUI: Update\nUI: Change Panel >> Home\n//UI: Front Panel State >> Open"  # UI: Initialize UI: Update UI: Change Panel >> Home //UI: Front Panel State >> Open
            # "Initialization Macro\n(This is called once, when the VI starts)"
            n100 = call <vilib>:"Add State(s) to Queue__jki_lib_state_machine.vi"("State(s) in Front (\"\")"="Data: Initialize\nInitialize Core Data\nEvents: Register", "State(s) in (\"\")"="Process: Sync", "State(s) at Back (\"\")"=w304) -> ("States Out"=w303:string)  [unwired: 12 in]
            n101 = call <vilib>:"Add State(s) to Queue__jki_lib_state_machine.vi"("State(s) in Front (\"\")"=w303, "State(s) in (\"\")"=w310) -> ("States Out"=w309:string)  [unwired: 13 in]
          }
          frame "Macro: Exit" {
            # "Exit Macro\n(This is called once, when the VI exits)"
            n102 = Unbundle By Name(w315) -> ("Core.Close Panel on Exit?"=w321:bool)
            n103 = Select(t="//UI: Front Panel State >> Close", s=w321, f="") -> (s? t:f=w318:string)
            n104 = call <vilib>:"Add State(s) to Queue__jki_lib_state_machine.vi"("State(s) in Front (\"\")"="Data: Cleanup\nEvents: Unregister", "State(s) in (\"\")"="Process: Sync", "State(s) at Back (\"\")"="Exit") -> ("States Out"=w312:string)  [unwired: 12 in]
            n105 = call <vilib>:"Add State(s) to Queue__jki_lib_state_machine.vi"("State(s) in (\"\")"=w318, "State(s) at Back (\"\")"=w312) -> ("States Out"=w317:string)  [unwired: 13 in]
            n106 = call <vilib>:"Add State(s) to Queue__jki_lib_state_machine.vi"("State(s) in Front (\"\")"=w317, "State(s) in (\"\")"=w324) -> ("States Out"=w323:string)  [unwired: 13 in]
          }
          frame "---------- Process ----------" {
            # "Template Separator\n(You can make a copy of, or modify, this frame)"
            n107 = call <vilib>:"Add State(s) to Queue__jki_lib_state_machine.vi"("State(s) in (\"\")"=w329) -> ("States Out"=w328:string)  [unwired: 14 in]
          }
          frame "Process: Sync" {
            n108 = Unbundle By Name(w337) -> ("Self Reference"=w333:refnum<class "GUI.lvclass">)
            n109 = call <vilib>:"WaitOnProcessSync.vi"("error in (no error)"=w332, "SMO"=w333) -> ("error out"=w331:errorcluster, "Don't run?"=w336:bool)  [unwired: 7 in, 1 out]
            n110 = Select(t="Data: Cleanup\nEvents: Unregister\nExit", s=w336, f="") -> (s? t:f=w330:string)
            n111 = call <vilib>:"Add State(s) to Queue__jki_lib_state_machine.vi"("State(s) in Front (\"\")"=w330, "State(s) in (\"\")"=w340) -> ("States Out"=w339:string)  [unwired: 13 in]
          }
          frame "---------- Events ----------" {
            # "Template Separator\n(You can make a copy of, or modify, this frame)"
            n112 = call <vilib>:"Add State(s) to Queue__jki_lib_state_machine.vi"("State(s) in (\"\")"=w345) -> ("States Out"=w344:string)  [unwired: 14 in]
          }
          frame "Events: Register" {
            n113 = Unbundle By Name(w372) -> ("Self Reference"=w363:refnum<class "GUI.lvclass">)
            n114 = call "GUI.GetPrivateEvents.vi"("GUI"=w363) -> ("error out"=w366:errorcluster, "Private Events"=w369:T9)  [unwired: 8 in, 1 out]
            n115 = call <vilib>:"ListDependencies.vi"("SMO in"=w363) -> ("error out"=w356:errorcluster, "[Dependencies]"=w362:refnum<class "SMO.lvclass">[])  [unwired: 7 in, 2 out]
            n116 = call <vilib>:"GetProtectedEvents.vi"("SMO"=w363) -> ("error out"=w368:errorcluster, "SMO Protected Events"=w370:T10)  [unwired: 8 in, 1 out]
            n117 = Index Array(array=w362) -> (element #1=w361:refnum<class "SMO.lvclass">, element #2=w355:refnum<class "SMO.lvclass">, element #3=w349:refnum<class "SMO.lvclass">)  [unwired: 3 in]
            n118 = To More Specific Class(target class=refnum<class "Home.lvclass"> refnum ("Home.lvclass"), reference=w349) -> (specific class reference=w348:refnum<class "Home.lvclass">)  [unwired: 1 in, 1 out]
            n119 = To More Specific Class(target class=refnum<class "Analyzer.lvclass"> refnum ("Analyzer.lvclass"), reference=w355) -> (specific class reference=w353:refnum<class "Analyzer.lvclass">)  [unwired: 1 in, 1 out]
            n120 = To More Specific Class(target class=refnum<class "DB2.lvclass"> refnum ("DB2.lvclass"), reference=w361) -> (specific class reference=w359:refnum<class "DB2.lvclass">)  [unwired: 1 in, 1 out]
            n121 = call "Home.GetPublicEvents.vi"("Home"=w348) -> ("error out"=w347:errorcluster, "SMO.Home Public Events"=w346:T11)  [unwired: 8 in, 1 out]
            n122 = call "Analyzer.GetPublicEvents.vi"("Analyzer"=w353) -> ("error out"=w352:errorcluster, "SMO.Analyzer Public Events"=w351:T12)  [unwired: 8 in, 1 out]
            n123 = call "DB2.GetPublicEvents.vi"("DB2"=w359) -> ("error out"=w357:errorcluster, "SMO.DB2 Public Events"=w358:T13)  [unwired: 8 in, 1 out]
            n124 = register-events(w370, w369, w358, w351, w346) -> (reference out=w371:refnum<event-registration>, error out=w365:errorcluster)  [unwired: 2 in]
            n125 = Merge Errors(w347, w352, w356, w357, w367, w368, w366, w365) -> (w364:errorcluster)
            n126 = call <vilib>:"Add State(s) to Queue__jki_lib_state_machine.vi"("State(s) in (\"\")"=w374) -> ("States Out"=w373:string)  [unwired: 14 in]
          }
          frame "Events: Unregister" {
            n127 = Unregister For Events(event registration refnum=w377, error in=w376) -> (error out=w375:errorcluster)
            n128 = call <vilib>:"Clear Errors.vi"("error in (no error)"=w375) -> ()  [unwired: 5 in, 2 out]
            n129 = call <vilib>:"Add State(s) to Queue__jki_lib_state_machine.vi"("State(s) in (\"\")"=w380) -> ("States Out"=w379:string)  [unwired: 14 in]
          }
          frame "---------- Action ----------" {
            n130 = call <vilib>:"Add State(s) to Queue__jki_lib_state_machine.vi"("State(s) in (\"\")"=w385) -> ("States Out"=w384:string)  [unwired: 14 in]
          }
          frame "Action: Get Settings" {
            n131 = Unbundle By Name(w393) -> ("Self Reference"=w392:refnum<class "GUI.lvclass">)
            n132 = call <vilib>:"ListDependencies.vi"("error in (no error)"=w386, "SMO in"=w392) -> ("error out"=w387:errorcluster, "[Dependencies]"=w391:refnum<class "SMO.lvclass">[])  [unwired: 6 in, 2 out]
            n133 = Index Array(array=w391, index=1) -> (element=w389:refnum<class "SMO.lvclass">)
            n134 = To More Specific Class(target class=refnum<class "Analyzer.lvclass"> refnum ("Analyzer.lvclass"), reference=w389, error in=w387) -> ()  [unwired: 2 out]
            n135 = call <vilib>:"Add State(s) to Queue__jki_lib_state_machine.vi"("State(s) in (\"\")"=w396) -> ("States Out"=w395:string)  [unwired: 14 in]
          }
          frame "Action: New Value" {
            n136 = Unbundle By Name(w401) -> ("Self Reference"=w400:refnum<class "GUI.lvclass">, "Value"=w399:T5)
            n137 = call "GUI.SetData.vi"("error in (no error)"=w398, "Value"=w399, "GUI"=w400) -> ("error out"=w397:errorcluster)  [unwired: 7 in, 1 out]
            n138 = call <vilib>:"Add State(s) to Queue__jki_lib_state_machine.vi"("State(s) in (\"\")"=w404) -> ("States Out"=w403:string)  [unwired: 14 in]
          }
          frame "Action: Notify UI Closed" {
            n139 = Unbundle By Name(w408) -> ("Self Reference"=w407:refnum<class "GUI.lvclass">)
            n140 = call <vilib>:"Hide.vi"("error in (no error)"=w406, "SMO.UI"=w407) -> ("error out"=w405:errorcluster)  [unwired: 8 in, 1 out]
            n141 = call <vilib>:"Add State(s) to Queue__jki_lib_state_machine.vi"("State(s) in (\"\")"=w411) -> ("States Out"=w410:string)  [unwired: 14 in]
          }
        }
      }
    }
    frame Error {
    }
  }
  n142 = call-parent "Process.vi"("error in (no error)"=w8, "SMO.UI"=w7) -> ("error out"=w5:errorcluster, "SMO.UI out"=→"GUI out":refnum<class "GUI.lvclass">)  [unwired: 8 in]
  n143 = Merge Errors(w5, w4) -> (→"error out":errorcluster)
